vi "WFDC Messenger Get Drift.vi"(11 "Error In":errorcluster) -> (4 "Status":T2, 8 "XYZ Drift":dbl[](array[numeric]), 13 "Cycle Sync":T1, 15 "Error Out":errorcluster)   [LabVIEW 2020]
uses:
  WFDC Controls/WFDC Status.ctl
  WFDC Controls/WFDC Cycle Pause.ctl
  WFDC Controls/WFDC External Sync.ctl
  WFDC Controls/WFDC Notifier Element.ctl
  WFDC Controls/WFDC Actions.ctl
  <vilib>/vision/Image Controls.llb/IMAQ Image.ctl
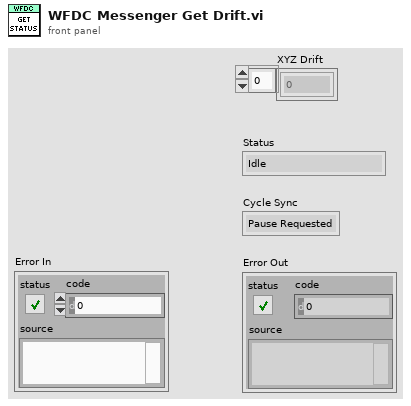
[diagram p1: front panel]
types:
  T1 = typedef "WFDC Cycle Pause.ctl" = enum16{"Pause Requested", "Paused", "Resume Requested", "Resumed"}
  T2 = typedef "WFDC Status.ctl" = enum16{"Idle", "Busy", "DC Active", "Error", "Canceled"}
  T3 = typedef "WFDC Notifier Element.ctl" = cluster{"WFDC Actions":T4, "Initial XYZ Positions":dbl[], "Ref Images":T5[], "Calibration (slope, inter)":dbl[], "Base Path":path, "Latest Scan Path":path, "Error":errorcluster, "XYZ Drift":dbl[]}
  T4 = typedef "WFDC Actions.ctl" = enum16{"Error Check", "Remote Start", "Move to Pos", "Pre Start Get Drift", "Pre Start Check Drift", "Pre Start Z Drift", "Pre Start XY Drift", "Pre Start ReFocus", "Setup New DC", "Setup Camera", "Get Ref Images", "Calc Calibration", "Switch Tabs", "Get Drift", "Z Drift", "XY Drift", "Start Cycle", "Stop DC", "Abort Remote", "Exit Loop", "Set Error", "Generate Calibration", "Quit"}
  T5 = typedef "IMAQ Image.ctl" = refnum<image>
  T6 = typedef "WFDC External Sync.ctl" = cluster{"Cycle Sync":T1, "Z Offset":dbl, "WFDC Status":T2}
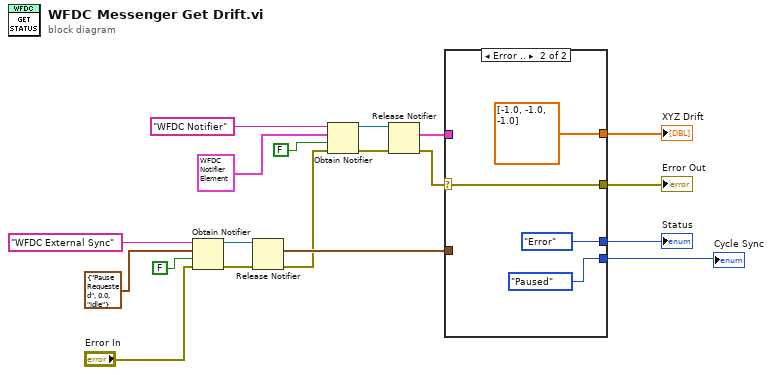
[diagram p0: block diagram]
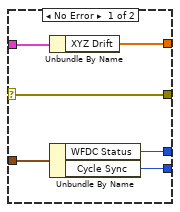
[diagram p2: hidden frame]
diagram:
  n1 = Obtain Notifier(name (unnamed)="WFDC External Sync", notification data type=T6 {"Cycle Sync"=enum."Pause Requested", "Z Offset"=0.0, "WFDC Status"=enum."Idle"} ("WFDC External Sync"), create if not found? (T)=FALSE, error in (no error)="Error In") -> (notifier out=w6:refnum<notifier>, error out=w4:errorcluster)  [unwired: 1 out]
  n2 = Release Notifier(notifier=w6, error in (no error)=w4) -> (last notification=w5:T6, error out=w3:errorcluster)  [unwired: 1 in, 1 out]
  n3 = Obtain Notifier(name (unnamed)="WFDC Notifier", notification data type=T3 {"WFDC Actions"=enum."Error Check", "Initial XYZ Positions"=[], "Ref Images"=[], "Calibration (slope, inter)"=[], "Base Path"=path "", "Latest Scan Path"=path "", "Error"={"status"=FALSE, "code"=0, "source"=""}, "XYZ Drift"=[]} ("WFDC Notifier Element"), create if not found? (T)=FALSE, error in (no error)=w3) -> (notifier out=w19:refnum<notifier>, error out=w18:errorcluster)  [unwired: 1 out]
  n4 = Release Notifier(notifier=w19, error in (no error)=w18) -> (last notification=w16:T3, error out=w17:errorcluster)  [unwired: 1 in, 1 out]
  n5 = case shown="Error .." w17 {
    selector: w17 -> [w23 w28]
    tunnel: w16 -> [w25 _]
    tunnel: [w24 dbl[] [-1.0, -1.0, -1.0] ("XYZ Drift")] -> w15
    tunnel: [w23 w28] -> w14
    tunnel: w5 -> [w22 _]
    tunnel: [w21 WFDC_Status."Error" ("WFDC Status")] -> w2
    tunnel: [w20 WFDC_Cycle_Pause."Paused" ("Cycle Sync")] -> w1
    frame No Error {
      n6 = Unbundle By Name(w25) -> ("XYZ Drift"=w24:dbl[])
      n7 = Unbundle By Name(w22) -> ("WFDC Status"=w21:T2, "Cycle Sync"=w20:T1)
    }
    frame Error {
    }
  }
  "Error Out" <- w14
  "XYZ Drift" <- w15
  "Status" <- w2
  "Cycle Sync" <- w1
